vi "Set Speed.vi"(8 "error in (no error)":errorcluster, 10 "FlowRate":dbl caption="Flow Rate (mL/min)", 11 "KNF Settings":T1={"VISA resource name"="", "Simulated?"=TRUE}) -> (0 "error out":errorcluster, 1 "Connection Error":bool, 3 "KNF Settings":T1={"VISA resource name"="", "Simulated?"=TRUE})   [LabVIEW 2018, in "KNF SIMDOS.lvlib"]
uses:
  KNF SIMDOS.lvlib
  Settings Cluster plus SIMDOS.ctl
  <vilib>/KNF LAB/Driver S/Lvlib/SIMLAB_driver_lvclass/SIMLAB_driver.lvclass
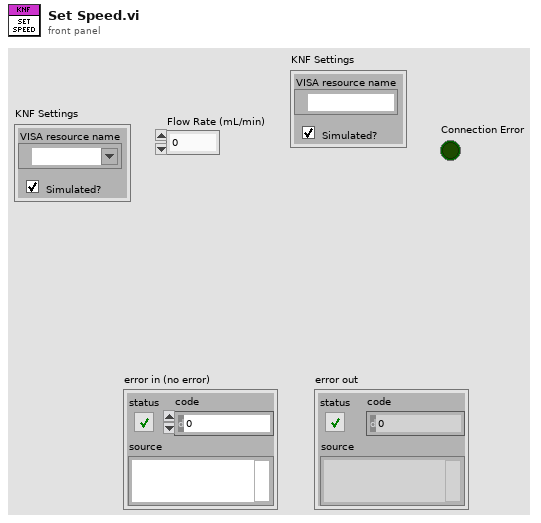
[diagram p1: front panel]
types:
  T1 = typedef "KNF SIMDOS.lvlib/Settings Cluster plus SIMDOS.ctl" = cluster{"VISA resource name":refnum<visa-resource-name>, "Simulated?":bool}
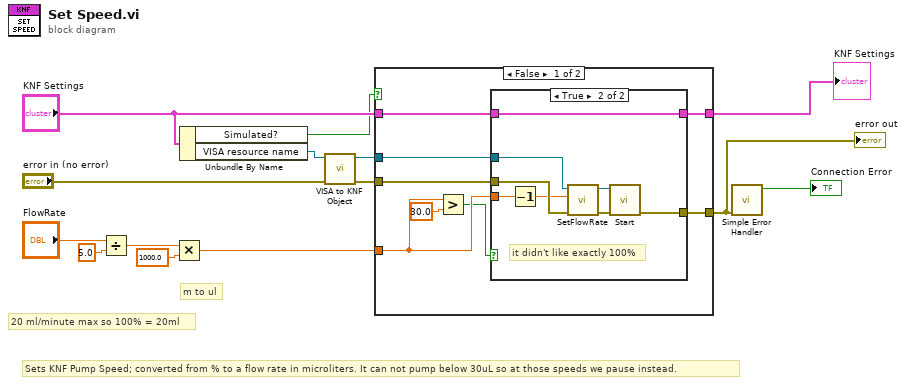
[diagram p0: block diagram]
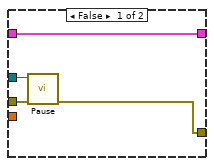
[diagram p2: hidden frame]
diagram:
  # "Sets KNF Pump Speed; converted from % to a flow rate in microliters. It can not pump below 30uL so at those speeds we pause instead."
  # "m to ul"
  # "20 ml/minute max so 100% = 20ml"
  n1 = Divide(x="FlowRate", y=5.0) -> (x/y=w1:dbl)
  n2 = Multiply(x=w1, y=1000.0) -> (x*y=w10:dbl)
  n3 = Unbundle By Name("KNF Settings") -> ("Simulated?"=w12:bool, "VISA resource name"=w7:refnum<visa-resource-name>)
  n4 = call "VISA to KNF Object.vi"("error in (no error)"="error in (no error)", "VISA resource name"=w7) -> ("error out"=w5:errorcluster, "SIMDOS out"=w6:refnum<class "SIMLAB_driver.lvclass">)  [unwired: 8 in]
  n5 = case shown="False" w12 {
    tunnel: [w22 w36] -> w9
    tunnel: w5 -> [w20 w36]
    tunnel: [w18 w35] -> w14
    tunnel: "KNF Settings" -> [w19 w35]
    tunnel: w6 -> [w21 _]
    tunnel: w10 -> [w17 _]
    frame False {
      n6 = Greater?(x=w17, y=30.0) -> (0:w16:bool)
      n7 = case shown="True" w16 {
        tunnel: [w24 w34] -> w22
        tunnel: w21 -> [w26 w33]
        tunnel: w20 -> [w25 w31]
        tunnel: w17 -> [_ w28]
        tunnel: w19 -> [w23 w29]
        tunnel: [w23 w29] -> w18
        frame False {
          n8 = call <vilib>:"Pause.vi"("error in (no error)"=w25, "SIMDOS in"=w26) -> ("error out"=w24:errorcluster)  [unwired: 8 in, 1 out]
        }
        frame True {
          # "it didn't like exactly 100%"
          n9 = Decrement(x=w28) -> (x-1=w27:dbl)
          n10 = call <vilib>:"SetFlowRate.vi"("error in (no error)"=w31, "FlowRate"=w27, "SIMDOS in"=w33) -> ("error out"=w30:errorcluster, "SIMDOS out"=w32:refnum<class "SIMLAB_driver.lvclass">)  [unwired: 7 in]
          n11 = call <vilib>:"Start.vi"("error in (no error)"=w30, "SIMDOS in"=w32) -> ("error out"=w34:errorcluster)  [unwired: 8 in, 1 out]
        }
      }
    }
    frame True {
    }
  }
  "error out" <- w9
  "KNF Settings" <- w14
  n12 = call <vilib>:"Simple Error Handler.vi"("error in (no error)"=w9) -> ("error?"=→"Connection Error":bool)  [unwired: 4 in, 4 out]
